vi "Close RFSG.vi"(8 "error in":errorcluster {"code" format="%.0x"}, 11 "instrument handle":refnum<k15>) -> (0 "error out":errorcluster {"code" format="%.0x"})   [LabVIEW 2018]
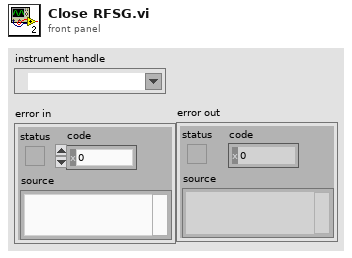
[diagram p1: front panel]
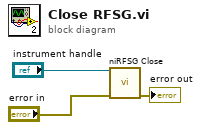
[diagram p0: block diagram]
diagram:
  n1 = call <instrlib>:"niRFSG Close.vi"("instrument handle"="instrument handle", "error in"="error in") -> ("error out"=→"error out":errorcluster)  [unwired: 13 in]
